vi "Wait Until Digital Edge.vi"(0 "Device ID":T4(ring), 2 "Wait Until":T2(ring), 5 "Module":T1(ring), 7 "Digital_Input":T3(ring), 11 "error in":errorcluster, 13 "Time Out (10)":dbl=10.0) -> (4 "Device ID Out":T4(ring), 15 "error out":errorcluster)   [LabVIEW 2010]
doc: "This VI waits until a user-defined digital edge is read."
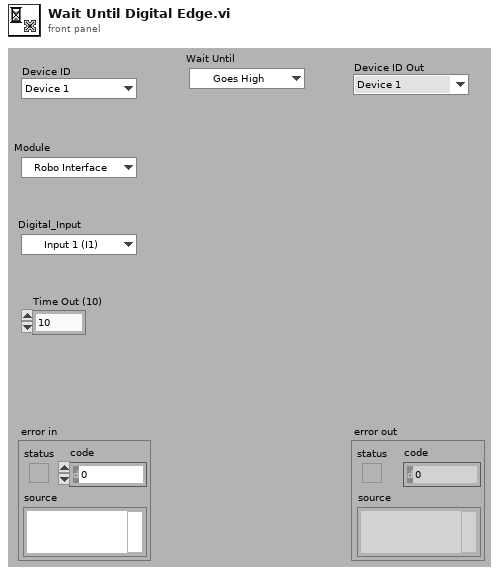
[diagram p1: front panel]
types:
  T1 = enum8{"Robo Interface", "Extension 1", "Extension 2", "Extension 3"}
  T2 = enum8{"Goes High", "Goes Low", "Goes High or Low"}
  T3 = enum8{"Input 1 (I1)", "Input 2 (I2)", "Input 3 (I3)", "Input 4 (I4)", "Input 5 (I5)", "Input 6 (I6)", "Input 7 (I7)", "Input 8 (I8)"}
  T4 = enum16{"Device 1", "Device 2", "Device 3", "Device 4", "Device 5", "Device 6", "Device 7", "Device 8"}
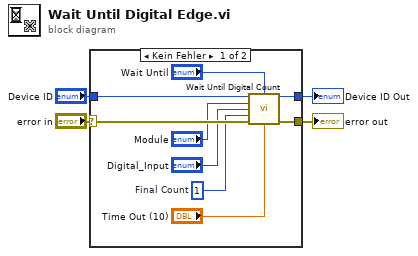
[diagram p0: block diagram]
diagram:
  n1 = case shown="Kein Fehler" "error in" {
    selector: "error in" -> [w9 w15]
    tunnel: [w10 w15] -> w3
    tunnel: "Device ID" -> [w12 w14]
    tunnel: [w11 w14] -> w1
    frame No Error {
      w5 = u32 1  # Final Count
      n2 = call "Wait Until Digital Count.vi"("Device ID"=w12, "Wait Until"="Wait Until", "Module"="Module", "Digital_Input"="Digital_Input", "Final Count"=w5, "error in"=w9, "Time Out (10)"="Time Out (10)") -> ("Device ID Out"=w11:T4, "error out"=w10:errorcluster)  [unwired: 7 out]
    }
    frame Error {
    }
  }
  "error out" <- w3
  "Device ID Out" <- w1
